vi "SD-Is Path and Not Empty.vi"(4 "path":path) -> (1 "Is Path and Not Empty?":bool)   [LabVIEW 2020]
doc: "Returns TRUE if <B>path</B> is any value other than <Not A Path> or an empty path. Otherwise, this VI returns FALSE."
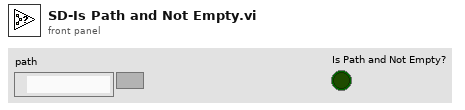
[diagram p1: front panel]
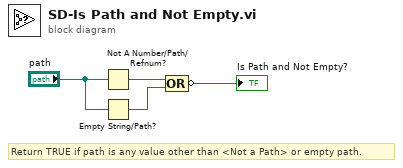
[diagram p0: block diagram]
diagram:
  # "Return TRUE if path is any value other than <Not a Path> or empty path."
  n1 = Not A Number/Path/Refnum?(number/path/refnum="path") -> (NaN/Path/Refnum?=w3:bool)
  n2 = Empty String/Path?(string/path="path") -> (empty?=w4:bool)
  n3 = Compound Arithmetic op=OR(w3, w4) -> (invert →"Is Path and Not Empty?":bool)
